vi "RectRegionConstraint_IsPoseInRegion.vi"(10 "statePose":T4={"TRANSLATION"={"X"=0.0, "Y"=0.0}, "ROTATION"={"VALUE"=0.0, "COS"=1.0, "SIN"=0.0}} {"ROTATION"."SIN" format="%13.4f"; "ROTATION"."COS" format="%13.4f"; "ROTATION"."VALUE" format="%13.4f"; "TRANSLATION"."Y" format="%14.3f"; "TRANSLATION"."X" format="%14.3f"}, 11 "RECT_REGION_CONSTRAINT":T1={"BottomLeftPoint"={"X"=0.0, "Y"=0.0}, "TopRightPoint"={"X"=0.0, "Y"=0.0}, "Constraint"=variant, "Constraint Type"=enum."DIFF DRIVE KINEMATICS"} {"TopRightPoint"."Y" format="%14.3f"; "TopRightPoint"."X" format="%14.3f"; "BottomLeftPoint"."Y" format="%14.3f"; "BottomLeftPoint"."X" format="%14.3f"}) -> (3 "PoseInRegion":bool)   [LabVIEW 2019, in "Trajectory_Library.lvlib"]
doc: "Determines if the robot pose is within the defined region.\n\nParameters:\n - Rectangular Region Constraint -- Constraint data cluster.\n - statePose - current traj state Pose\n\nReturns\n - PoseInRegion -- TRUE if pose is within the region."
uses:
  Trajectory_Library.lvlib
  TypeDef/TRANSLATION2D.ctl
  TypeDef/ROTATION2D.ctl
  TypeDef/POSE2D.ctl
  Enum/TRAJ_CONSTRAINT_TYPES_ENUM.ctl
  TypeDef/TRAJ_CONSTRAINT_RECT_REGION.ctl
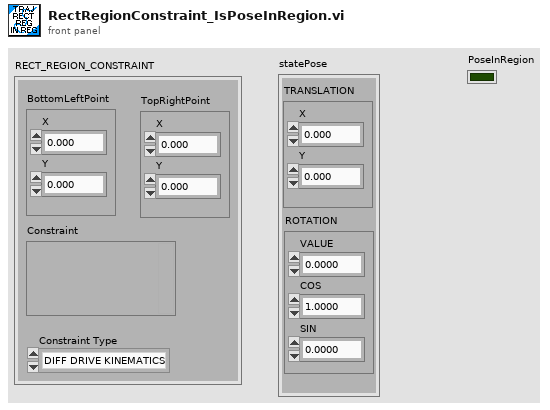
[diagram p1: front panel]
types:
  T1 = typedef "Trajectory_Library.lvlib/TRAJ_CONSTRAINT_RECT_REGION.ctl" = cluster{"BottomLeftPoint":T2, "TopRightPoint":T2, "Constraint":variant, "Constraint Type":T3}
  T2 = typedef "Trajectory_Library.lvlib/TRANSLATION2D.ctl" = cluster{"X":dbl, "Y":dbl}
  T3 = typedef "Trajectory_Library.lvlib/TRAJ_CONSTRAINT_TYPES_ENUM.ctl" = enum16{"UNDEFINED", "DIFF DRIVE KINEMATICS", "DIFF DRIVE VOLTAGE", "CENTRIPITAL ACCEL", "MECA DRIVE KINEMATICS", "SWERVE DRIVE KINEMATICS", "MAXIMUM VELOCITY", "ELLIPTICAL REGION", "RECTANGULAR REGION"}
  T4 = typedef "Trajectory_Library.lvlib/POSE2D.ctl" = cluster{"TRANSLATION":T2, "ROTATION":T5}
  T5 = typedef "Trajectory_Library.lvlib/ROTATION2D.ctl" = cluster{"VALUE":dbl, "COS":dbl, "SIN":dbl}
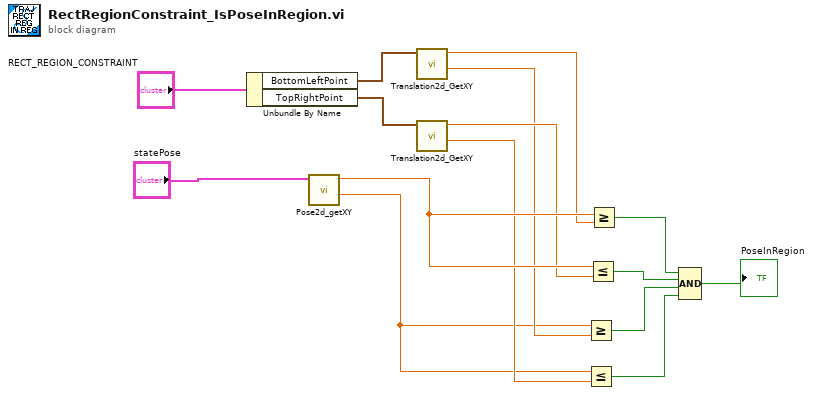
[diagram p0: block diagram]
diagram:
  n1 = Unbundle By Name("RECT_REGION_CONSTRAINT") -> ("BottomLeftPoint"=w14:T2, "TopRightPoint"=w13:T2)
  n2 = call "Pose2d_getXY.vi"("in POSE"="statePose") -> ("Y"=w6:dbl, "X"=w11:dbl)  [unwired: 9 in]
  n3 = call "Translation2d_GetXY.vi"("In Translation"=w14) -> ("Y"=w8:dbl, "X"=w10:dbl)  [unwired: 9 in]
  n4 = call "Translation2d_GetXY.vi"("In Translation"=w13) -> ("Y"=w7:dbl, "X"=w9:dbl)  [unwired: 9 in]
  n5 = Greater Or Equal?(x=w6, y=w8) -> (x >= y?=w3:bool)
  n6 = Less Or Equal?(x=w6, y=w7) -> (x <= y?=w2:bool)
  n7 = Less Or Equal?(x=w11, y=w9) -> (x <= y?=w4:bool)
  n8 = Greater Or Equal?(x=w11, y=w10) -> (x >= y?=w5:bool)
  n9 = Compound Arithmetic op=AND(w5, w4, w3, w2) -> (→"PoseInRegion":bool)
